vi "Relocate Splitter Posistion.vi"(8 "Error in":errorcluster caption="Error in (no error)", 10 "Array":refnum<vi>[](array[refnum]), 11 "Splitter in":refnum<vi>) -> (0 "Error out":errorcluster)   [LabVIEW 2017]
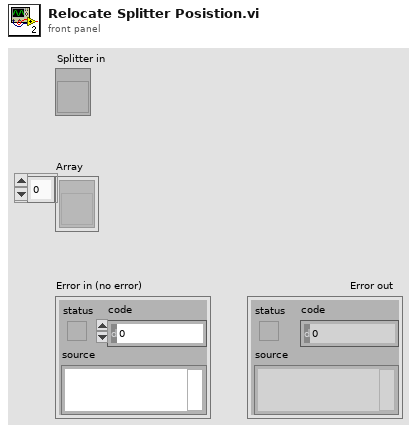
[diagram p1: front panel]
types:
  T1 = typedef "LVPositionTypeDef.ctl" = cluster{"Left":i32, "Top":i32}
  T2 = typedef "LVRectTypeDef.ctl" = cluster{"Left":i16, "Top":i16, "Right":i16, "Bottom":i16}
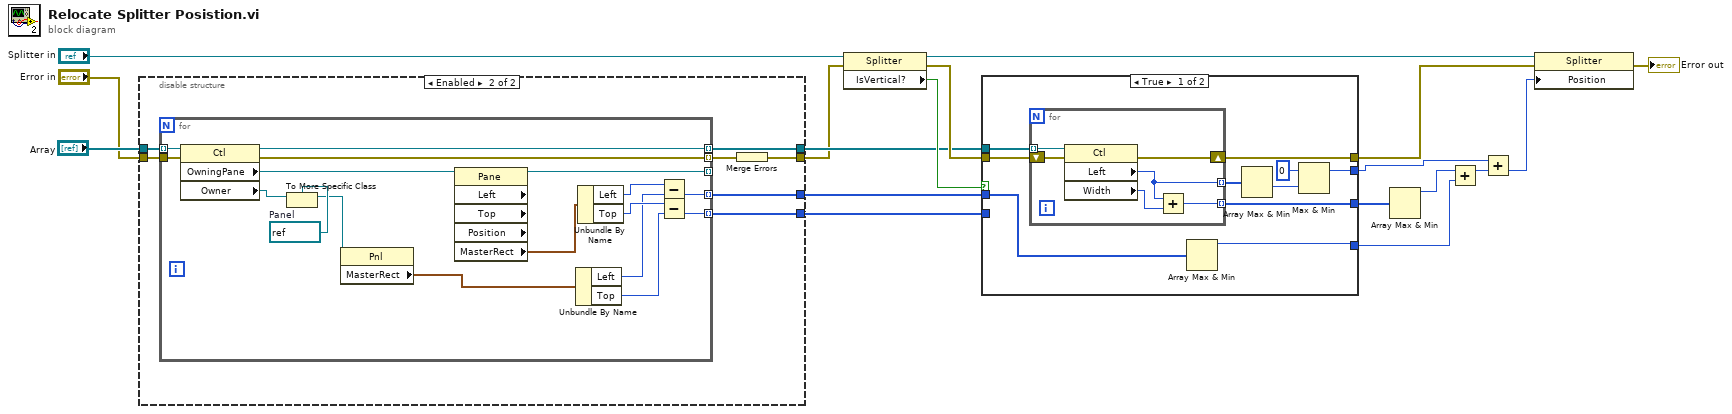
[diagram p0: block diagram]
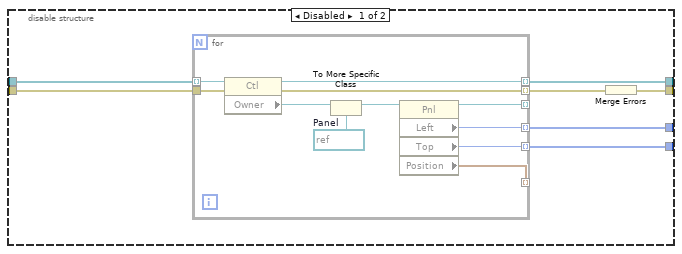
[diagram p2: hidden frame]
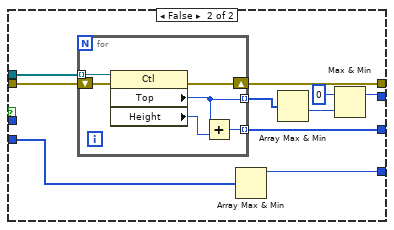
[diagram p3: hidden frame]
diagram:
  n1 = disable-structure shown="Enabled" {
    disable-tunnel: [w25 w43] -> w11
    disable-tunnel: "Array" -> [w24 w42]
    disable-tunnel: "Error in" -> [w23 w41]
    disable-tunnel: [w21 w39] -> w8
    disable-tunnel: [w20 w38] -> w7
    disable-tunnel: [w19 w37] -> w6
    frame Disabled {
      n2 = for {
        tunnel: [w35] -> w25 mode=indexing
        tunnel: w24 -> [w36] mode=indexing
        tunnel: [w34] -> _ mode=indexing
        tunnel: [w33] -> w20 mode=indexing
        tunnel: [w32] -> w19 mode=indexing
        tunnel: w23 -> [w31]
        tunnel: [w30] -> w22 mode=indexing
        tunnel: [w29] -> _ mode=indexing
        w26 = refnum<vi> refnum  # Panel
        n3 = property class="Ctl"(reference=w36, error in=w31) -> (reference out=w35:refnum<vi>, error out=w30:errorcluster, "Owner"=w27:refnum<vi>)
        n4 = To More Specific Class(target class=w26, reference=w27) -> (specific class reference=w28:refnum<vi>)  [unwired: 1 in, 1 out]
        n5 = property class="Pnl"(reference=w28) -> (reference out=w34:refnum<vi>, "Left"=w33:i32, "Top"=w32:i32, "Position"=w29:T1)  [unwired: 1 in, 1 out]
      }
      n6 = Merge Errors(w22) -> (w21:errorcluster)
    }
    frame Enabled {
      n7 = for {
        tunnel: [w59] -> w43 mode=indexing
        tunnel: w42 -> [w60] mode=indexing
        tunnel: [w58] -> _ mode=indexing
        tunnel: [w52] -> w38 mode=indexing
        tunnel: [w53] -> w37 mode=indexing
        tunnel: w41 -> [w57]
        tunnel: [w56] -> w40 mode=indexing
        w49 = refnum<vi> refnum  # Panel
        n8 = property class="Ctl"(reference=w60, error in=w57) -> (reference out=w59:refnum<vi>, error out=w56:errorcluster, "OwningPane"=w55:refnum<vi>, "Owner"=w48:refnum<vi>)
        n9 = To More Specific Class(target class=w49, reference=w48) -> (specific class reference=w47:refnum<vi>)  [unwired: 1 in, 1 out]
        n10 = property class="Pnl"(reference=w47) -> ("MasterRect"=w46:T2)  [unwired: 1 in, 2 out]
        n11 = property class="Pane" props=["Left", "Top", "Position", "MasterRect"](reference=w55) -> (reference out=w58:refnum<vi>, "MasterRect"=w54:T2)  [unwired: 1 in, 4 out]
        n12 = Unbundle By Name(w46) -> ("Left"=w45:i16, "Top"=w44:i16)
        n13 = Unbundle By Name(w54) -> ("Left"=w51:i16, "Top"=w50:i16)
        n14 = Subtract(x=w51, y=w45) -> (x-y=w52:i16)
        n15 = Subtract(x=w50, y=w44) -> (x-y=w53:i16)
      }
      n16 = Merge Errors(w40) -> (w39:errorcluster)
    }
  }
  n17 = property class="Splitter"(reference="Splitter in", error in=w8) -> (reference out=w15:refnum<vi>, error out=w17:errorcluster, "IsVertical?"=w16:bool)
  n18 = case shown="True" w16 {
    tunnel: w11 -> [w70 w86]
    tunnel: [w69 w85] -> w13
    tunnel: w17 -> [w67 w84]
    tunnel: [w68 w83] -> w18
    tunnel: w7 -> [w66 _]
    tunnel: w6 -> [_ w82]
    tunnel: [w65 w81] -> w3
    tunnel: [w62 w77] -> w1
    frame True {
      n19 = for {
        tunnel: w70 -> [w76] mode=indexing
        tunnel: [w74] -> w69 mode=indexing
        shift-right: [w73] -> w68
        shift-left: w67 -> [w72]
        tunnel: [w71] -> w61 mode=indexing
        n20 = property class="Ctl"(reference=w76, error in=w72) -> (error out=w73:errorcluster, "Left"=w71:i32, "Width"=w75:u32)  [unwired: 1 out]
        n21 = Add(x=w71, y=w75) -> (x+y=w74:u32)
      }
      n22 = Array Max & Min(array=w66) -> (max value=w65:i16)  [unwired: 3 out]
      n23 = Array Max & Min(array=w61) -> (min value=w64:i32)  [unwired: 3 out]
      n24 = Max & Min(x=0, y=w64) -> (max(x,y)=w62:i32)  [unwired: 1 out]
    }
    frame False {
      n25 = for {
        tunnel: w86 -> [w92] mode=indexing
        tunnel: [w90] -> w85 mode=indexing
        shift-right: [w88] -> w83
        shift-left: w84 -> [w89]
        tunnel: [w87] -> w80 mode=indexing
        n26 = property class="Ctl"(reference=w92, error in=w89) -> (error out=w88:errorcluster, "Top"=w87:i32, "Height"=w91:u32)  [unwired: 1 out]
        n27 = Add(x=w87, y=w91) -> (x+y=w90:u32)
      }
      n28 = Array Max & Min(array=w82) -> (max value=w81:i16)  [unwired: 3 out]
      n29 = Array Max & Min(array=w80) -> (min value=w79:i32)  [unwired: 3 out]
      n30 = Max & Min(x=0, y=w79) -> (max(x,y)=w77:i32)  [unwired: 1 out]
    }
  }
  n31 = Array Max & Min(array=w13) -> (max value=w4:u32)  [unwired: 3 out]
  n32 = Add(x=w4, y=w3) -> (x+y=w5:u32)
  n33 = Add(x=w1, y=w5) -> (x+y=w2:u32)
  n34 = property class="Splitter"(reference=w15, error in=w18, "Position"=w2) -> (error out=→"Error out":errorcluster)  [unwired: 1 out]
